vi "Reacquire Target In FOV.vi"(0 "System of Reference Interface":T1, 5 "Focus and Tracking":T2, 11 "error in (no error)":errorcluster) -> (4 "Optical Coordinates [um]":cluster{"X":dbl, "Y":dbl, "Z":dbl}, 6 "Focus Ok":bool, 8 "Scope Error":bool, 15 "error out":errorcluster)   [LabVIEW 2012]
uses:
  <vilib>/Analysis/Matrix/Datatypes/RealMatrix.ctl
  Targeting Unit.lvlib
  <vilib>/Analysis/Matrix/NI_Matrix.lvlib
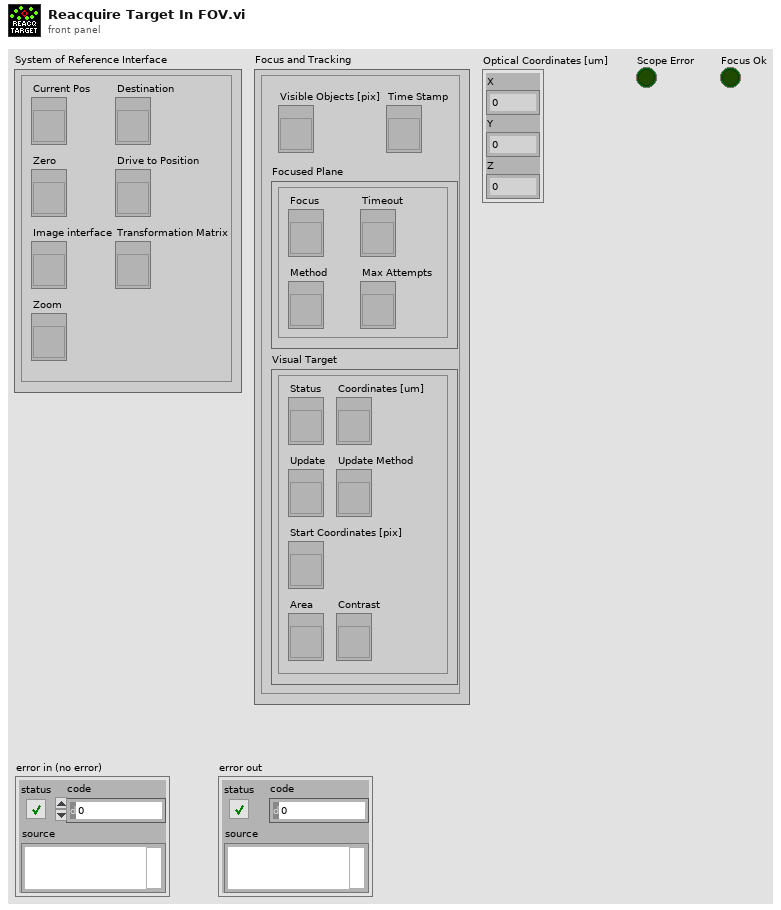
[diagram p1: front panel]
types:
  T1 = cluster{"Current Pos":refnum<vi>, "Image interface":refnum<vi>, "Transformation Matrix":refnum<vi>, "Zero":refnum<vi>, "Destination":refnum<vi>, "Drive to Position":refnum<vi>, "Zoom":refnum<vi>}
  T2 = cluster{"Focused Plane":cluster{"Focus":refnum<vi>, "Timeout":refnum<vi>, "Max Attempts":refnum<vi>, "Method":refnum<vi>}, "Time Stamp":refnum<vi>, "Visual Target":cluster{"Coordinates [um]":refnum<vi>, "Status":refnum<vi>, "Update":refnum<vi>, "Update Method":refnum<vi>, "Start Coordinates [pix]":refnum<vi>, "Area":refnum<vi>, "Contrast":refnum<vi>}, "Visible Objects [pix]":refnum<vi>}
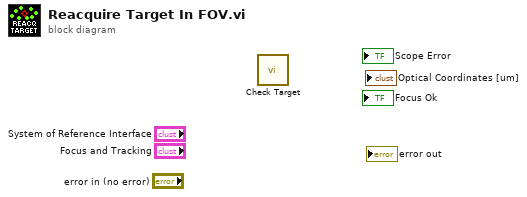
[diagram p0: block diagram]
diagram:
  n1 = call "Check Target.vi"() -> ()  [unwired: 5 in, 7 out]
